vi "Arm(CommitSettings).vi"(7 "Arm?":bool=TRUE, 8 "error in":errorcluster, 11 "FPGA VI Reference In":refnum<k20>) -> (0 "error out":errorcluster, 3 "FPGA VI Reference Out":refnum<k20>)   [LabVIEW 2020]
uses:
  <vilib>/Utility/error.llb/Error Cluster From Error Code.vi
  <vilib>/rvi/errors/niLvFpgaAdjustHostInterfaceError.vi
  <vilib>/rvi/interface/nirviReadWriteControl/nirviReadWriteControl.xnode
  NiFpgaLv.dll
  <vilib>/rvi/interface/Simulation/niFpgaSimulationCallBeginRW.vi
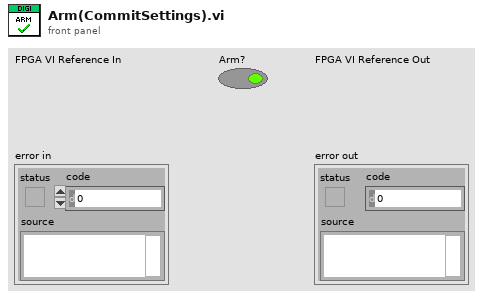
[diagram p1: front panel]
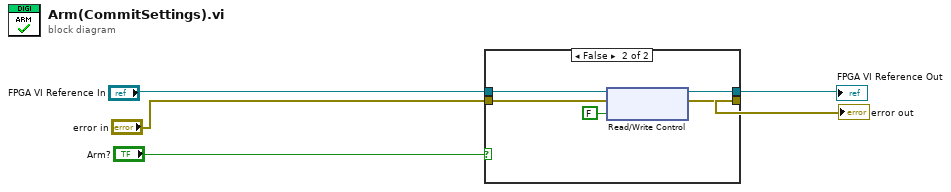
[diagram p0: block diagram]
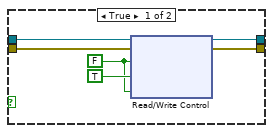
[diagram p2: hidden frame]
diagram:
  n1 = case shown="False" "Arm?" {
    tunnel: "FPGA VI Reference In" -> [w11 w16]
    tunnel: "error in" -> [w10 w15]
    tunnel: [w9 w14] -> w5
    tunnel: [w8 w13] -> w3
    frame True {
      w6 = FALSE ("Arm Trigger")
      n2 = xnode "Read/Write Control"("FPGA VI Reference In"=w11, "error in"=w10, "Arm Trigger"=w6, "Arm Trigger"=TRUE, "Arm Trigger"=w6) -> ("FPGA VI Reference Out"=w9:refnum<k20>, "error out"=w8:errorcluster)
    }
    frame False {
      n3 = xnode "Read/Write Control"("FPGA VI Reference In"=w16, "error in"=w15, "Arm Trigger"=FALSE) -> ("FPGA VI Reference Out"=w14:refnum<k20>, "error out"=w13:errorcluster)
    }
  }
  "error out" <- w3
  "FPGA VI Reference Out" <- w5
